vi "Last Character in String.vi"(0 "Input  String (empty)":string) -> (1 "Last Character":string, 2 "Rest of String":string)   [LabVIEW 2020, in "Associated Research 78XX Series.lvlib"]
doc: "This utility vi breaks off the last character of a string and also returns the remaining portion of the string."
uses:
  <instrlib>/Associated Research 78XX Series/Associated Research 78XX Series.lvlib
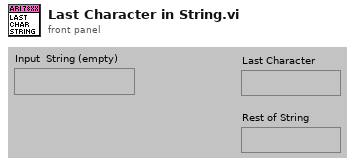
[diagram p1: front panel]
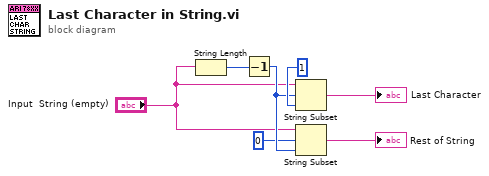
[diagram p0: block diagram]
diagram:
  n1 = String Length(string="Input  String (empty)") -> (length=w6:i32)
  n2 = Decrement(x=w6) -> (x-1=w4:i32)
  n3 = String Subset(string="Input  String (empty)", offset (0)=w4, length (rest)=1) -> (substring=→"Last Character":string)
  n4 = String Subset(string="Input  String (empty)", offset (0)=0, length (rest)=w4) -> (substring=→"Rest of String":string)
